vi "Open.vi"(6 "wait for reply (T)":bool=TRUE, 8 "error in":errorcluster, 10 "Resource":string) -> (0 "error out":errorcluster, 1 "timed out?":bool)   [LabVIEW 2021, in "PS.lvlib"]
doc: "_____\nCreated using DQMH Event Scripter 6.1.0.128."
uses:
  PS.lvlib
  Open Argument--cluster.ctl
  Open (Reply Payload)--cluster.ctl
  <vilib>/DQMH Consortium/Lumos API/Libraries/SDV API/SDV API.lvlib
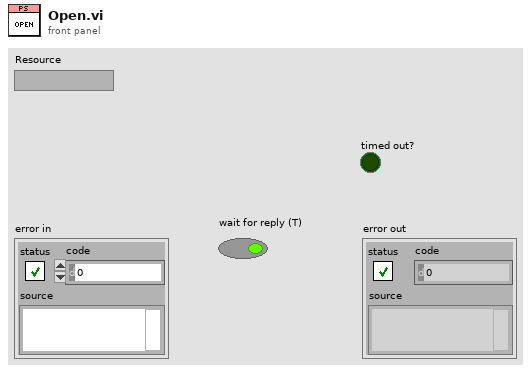
[diagram p1: front panel]
types:
  T1 = typedef "PS.lvlib/Open Argument--cluster.ctl" = cluster{"Resource":string, "Wait Notifier":refnum<notifier>, "wait for reply":bool}
  T2 = typedef "PS.lvlib/Request Events--cluster.ctl" = cluster{"Stop Module":refnum<user-event>, "Show Panel":refnum<user-event>, "Hide Panel":refnum<user-event>, "Get Module Execution Status":refnum<user-event>, "Show Diagram":refnum<user-event>, "Set Power Supply":refnum<user-event>, "Set Voltage":refnum<user-event>, "Set Current":refnum<user-event>, "Set Output":refnum<user-event>, "Open":refnum<user-event>, "Close":refnum<user-event>, "Get PS Data":refnum<user-event>, "Load in SubPane":refnum<user-event>, "UnLoad SubPane":refnum<user-event>}
  T3 = typedef "PS.lvlib/Open (Reply Payload)--cluster.ctl" = cluster{"error":errorcluster}
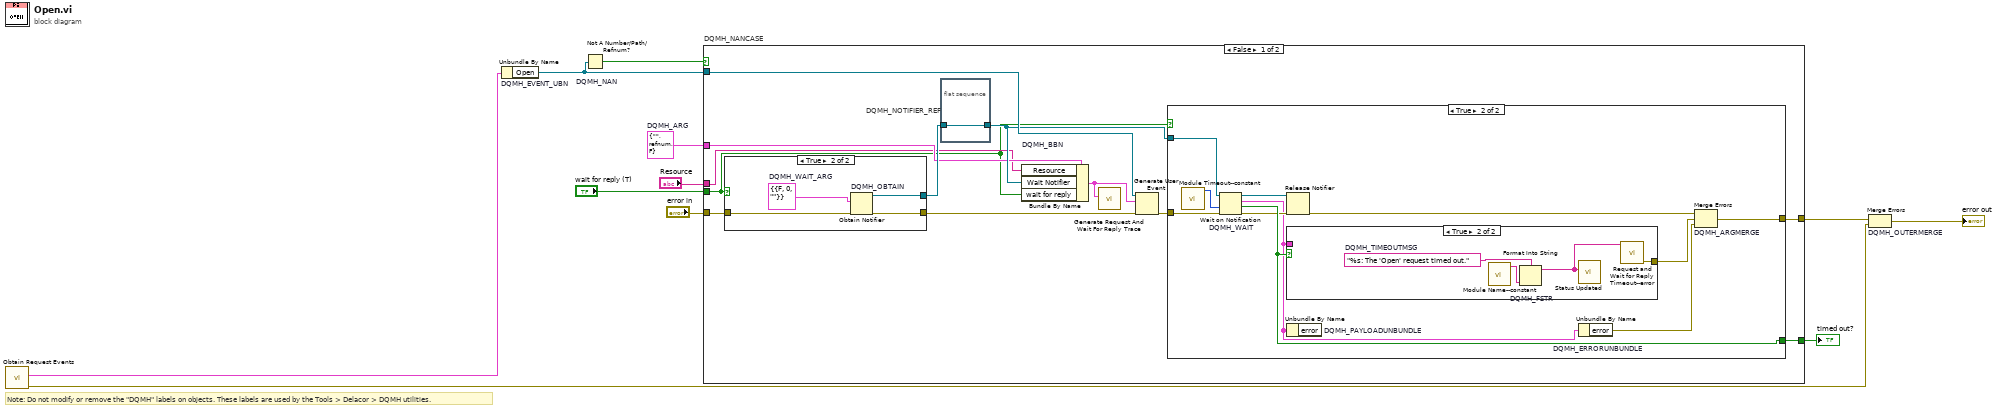
[diagram p0: block diagram]
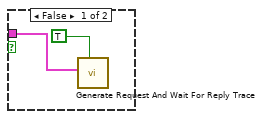
[diagram p3: hidden frame]
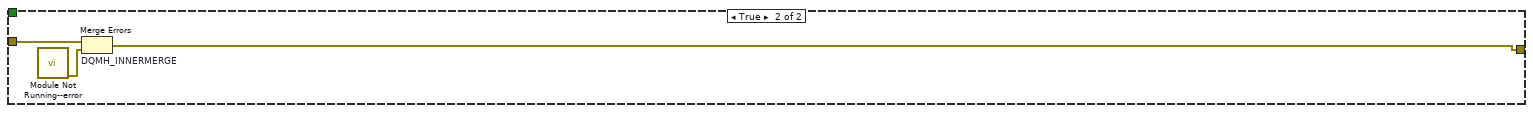
[diagram p5: hidden frame]
diagram:
  w5 = T1 {"Resource"="", "Wait Notifier"=refnum, "wait for reply"=FALSE}  # DQMH_ARG
  # "Note: Do not modify or remove the \"DQMH\" labels on objects. These labels are used by the Tools > Delacor > DQMH utilities."
  n1 = call "Obtain Request Events.vi"() -> ("error out"=w2:errorcluster, "PS Request Events"=w1:T2)  [unwired: 10 in]
  n2 = Unbundle By Name "DQMH_EVENT_UBN"(w1) -> ("Open"=w9:refnum<user-event>)
  n3 = Not A Number/Path/Refnum? "DQMH_NAN"(number/path/refnum=w9) -> (NaN/Path/Refnum?=w8:bool)
  n4 = case "DQMH_NANCASE" shown="False" w8 {
    tunnel: "error in" -> [w23 w50]
    tunnel: w9 -> [w21 _]
    tunnel: [w18 w49] -> w6
    tunnel: [w19 _] -> w7
    tunnel: w5 -> [w14 _]
    tunnel: "Resource" -> [w13 _]
    tunnel: "wait for reply (T)" -> [w12 _]
    frame False {
      n5 = case shown="True" w12 {
        tunnel: w23 -> [w43 w47]
        tunnel: [w43 w46] -> w20
        tunnel: [_ w44] -> w16
        frame False {
        }
        frame True {
          w45 = T3 {"error"={"status"=FALSE, "code"=0, "source"=""}}  # DQMH_WAIT_ARG
          n6 = Obtain Notifier "DQMH_OBTAIN"(notification data type=w45, error in (no error)=w47) -> (notifier out=w44:refnum<notifier>, error out=w46:errorcluster)  [unwired: 2 in, 1 out]
        }
      }
      n7 = flat-sequence "DQMH_NOTIFIER_REF" {
        tunnel: w16 -> [w24]
        tunnel: [w24] -> w15
        frame #0 {
        }
      }
      n8 = Bundle By Name "DQMH_BBN"(cluster=w14, "Resource"=w13, "Wait Notifier"=w15, "wait for reply"=w12) -> (w17:T1)
      n9 = call <vilib>:"Generate Request And Wait For Reply Trace.vi"("Payload"=w17) -> ()  [unwired: 10 in, 1 out]
      n10 = Generate User Event(user event=w21, event data cluster=w17, error in=w20) -> (error out=w22:errorcluster)  [unwired: 1 in, 1 out]
      n11 = case shown="True" w12 {
        tunnel: w22 -> [w25 w36]
        tunnel: w15 -> [_ w35]
        tunnel: [_ w33] -> w19
        tunnel: [w25 w32] -> w18
        frame False {
        }
        frame True {
          n12 = call "Module Timeout--constant.vi"() -> ("Module Timeout"=w27:i32)  [unwired: 11 in]
          n13 = Wait on Notification "DQMH_WAIT"(notifier=w35, timeout in ms (-1)=w27, error in (no error)=w36) -> (notifier out=w34:refnum<notifier>, notification=w26:T3, timed out?=w33:bool, error out=w31:errorcluster)  [unwired: 1 in]
          n14 = Release Notifier(notifier=w34, error in (no error)=w31) -> (error out=w30:errorcluster)  [unwired: 1 in, 2 out]
          n15 = case shown="True" w33 {
            tunnel: [_ w40] -> w28
            tunnel: w26 -> [w37 _]
            frame False {
              n16 = call <vilib>:"Generate Request And Wait For Reply Trace.vi"("Reply (F)"=TRUE, "Payload"=w37) -> ()  [unwired: 9 in, 1 out]
            }
            frame True {
              w42 = "%s: The 'Open' request timed out."  # DQMH_TIMEOUTMSG
              n17 = call "Module Name--constant.vi"() -> ("Module Name"=w39:string)  [unwired: 11 in]
              n18 = Format Into String "DQMH_FSTR"(format string=w42, w39) -> (resulting string=w41:string)  [unwired: 2 in, 1 out]
              n19 = call "Status Updated.vi"("Status"=w41) -> ()  [unwired: 10 in, 1 out]
              n20 = call "Request and Wait for Reply Timeout--error.vi"("Error Message"=w41) -> ("error out"=w40:errorcluster)  [unwired: 10 in]
            }
          }
          n21 = Unbundle By Name "DQMH_PAYLOADUNBUNDLE"(w26) -> ()  [unwired: 1 out]
          n22 = Unbundle By Name "DQMH_ERRORUNBUNDLE"(w26) -> ("error"=w29:errorcluster)
          n23 = Merge Errors "DQMH_ARGMERGE"(w30, w28, w29) -> (w32:errorcluster)
        }
      }
    }
    frame True {
      n24 = call "Module Not Running--error.vi"() -> ("error out"=w48:errorcluster)  [unwired: 11 in]
      n25 = Merge Errors "DQMH_INNERMERGE"(w50, w48) -> (w49:errorcluster)
    }
  }
  "timed out?" <- w7
  n26 = Merge Errors "DQMH_OUTERMERGE"(w6, w2) -> (→"error out":errorcluster)
